vi "CreateUserEvent.vi"(8 "error in (no error)":errorcluster caption="错误输入（无错误）", 11 "事件消息":cluster{"事件名":string, "事件数据":string}) -> (0 "error out":errorcluster caption="错误输出", 2 "用户事件引用句柄":refnum<user-event>, 3 "用户事件注册引用句柄":refnum<event-registration>)   [LabVIEW 2018]
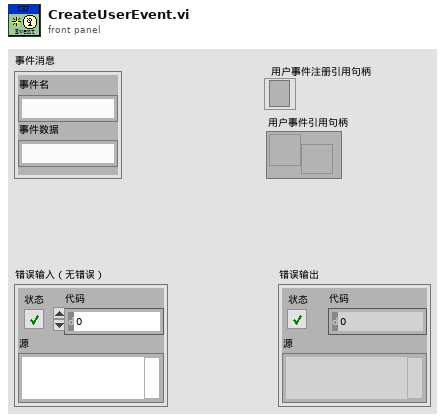
[diagram p1: front panel]
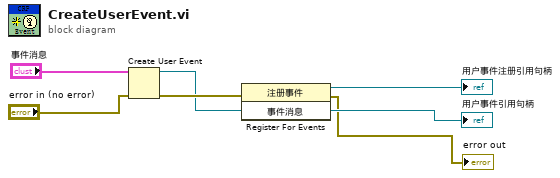
[diagram p0: block diagram]
diagram:
  n1 = Create User Event(user event datatype="事件消息", error in="error in (no error)") -> (user event=w2:refnum<user-event>, error out=w4:errorcluster)
  "用户事件引用句柄" <- w2
  n2 = register-events(error in=w4, w2) -> (reference out=→"用户事件注册引用句柄":refnum<event-registration>, error out=→"error out":errorcluster)  [unwired: 1 in]
